vi "ApplyFloatFormat.vi"(5 "Format for Real Values":string="%_3g", 9 "Values":variant[](array[variant])) -> (3 "Values Out":variant[](array[variant]))   [LabVIEW 2017]
panel:
  # "LVHDF5 Toolkit\nCopyright (c) 2005-2013 by Jason D. Sommerville\nCopyright (c) 2014 by UPVI, LLC.\n\nThis use and distribution of this file is governed by the terms found in \nLICENSE.txt distributed with this toolkit and installed at\n <user.lib>\\_lvhdf5\\LICENSE.txt"
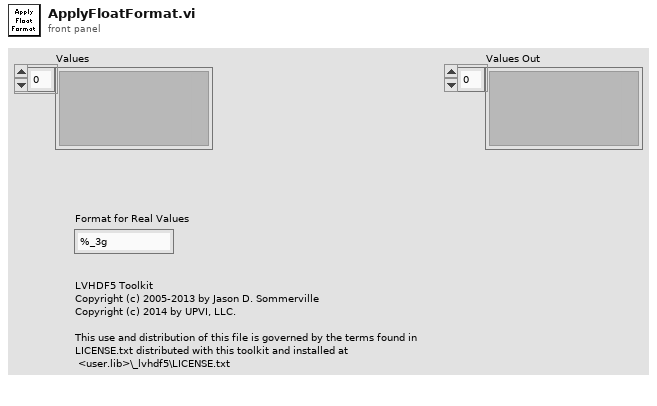
[diagram p1: front panel]
types:
  T1 = typedef "Type Descriptor Enumeration__ogtk.ctl" = enum8{"<Null>", "I8", "I16", "I32", "I64", "U8", "U16", "U32", "U64", "SGL", "DBL", "EXT", "CSG", "CDB", "CXT", "0x0F", "0x10", "0x11", "0x12", "0x13", "0x14", "Enum U8", "Enum U16", "Enum U32", "Enum U64", "SGL PQ", "DBL PQ", "EXT PQ", "CSG PQ", "CDB PQ", "CXT PQ", "0x1F", "0x20", "Boolean", "0x22", "0x23", "0x24", "0x25", "0x26", "0x27", "0x28", "0x29", "0x2A", "0x2B", "0x2C", "0x2D", "0x2E", "0x2F", "String", "0x31", "Path", "Pict", "0x34", "0x35", "0x36", "DAQ", "0x38", "0x39", "0x3A", "0x3B", "0x3C", "0x3D", "0x3E", "0x3F", "Array", "0x41", "0x42", "0x43", "0x44", "0x45", "0x46", "0x47", "0x48", "0x49", "0x4A", "0x4B", "0x4C", "0x4D", "0x4E", "0x4F", "Cluster", "0x51", "0x52", "Variant", "Waveform", "0x55", "0x56", "0x57", "0x58", "0x59", "0x5A", "0x5B", "0x5C", "0x5D", "0x5E", "0x5F", "0x60", "0x61", "0x62", "0x63", "0x64", "0x65", "0x66", "0x67", "0x68", "0x69", "0x6A", "0x6B", "0x6C", "0x6D", "0x6E", "0x6F", "Refnum"}
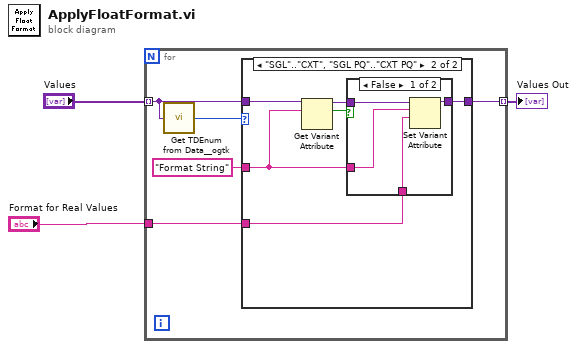
[diagram p0: block diagram]
diagram:
  n1 = for {
    tunnel: "Values" -> [w8] mode=indexing
    tunnel: "Format for Real Values" -> [w6]
    tunnel: [w5] -> w1 mode=indexing
    n2 = call <userlib>:"Get TDEnum from Data__ogtk.vi"("Data"=w8) -> ("Type Descriptor Enumeration"=w7:T1)  [unwired: 4 in]
    n3 = case shown="\"SGL\"..\"CXT\", \"SGL PQ\"..\"CXT PQ\"" w7 {
      tunnel: w8 -> [w9 w13]
      tunnel: w6 -> [_ w15]
      tunnel: [w9 w14] -> w5
      tunnel: "Format String" ("name") -> [_ w10]
      frame "<Null>", Default {
      }
      frame "SGL".."CXT", "SGL PQ".."CXT PQ" {
        n4 = Get Variant Attribute(Variant=w13, name=w10) -> (duplicate Variant=w12:variant, found=w11:bool)  [unwired: 2 in, 2 out]
        n5 = case shown="False" w11 {
          tunnel: w15 -> [w19 _]
          tunnel: [w18 w20] -> w14
          tunnel: w12 -> [w17 w20]
          tunnel: w10 -> [w16 _]
          frame False {
            n6 = Set Variant Attribute(Variant=w17, name=w16, value=w19) -> (Variant out=w18:variant)  [unwired: 1 in, 2 out]
          }
          frame True {
          }
        }
      }
    }
  }
  "Values Out" <- w1
